vi "ThreadCfg - Read TxPkt Config.vi"(8 "error in (no error)":errorcluster, 11 "Node Ptr In":T4 format="%.0x") -> (0 "error out":errorcluster, 2 "threadOptions":T1 {"pclDecimation" max=16 step=1; "loopPeriod" max=16 step=1; "targetPriority" min=-2 max=16 step=1; "targetProcessor" min=-2 max=16 step=1}, 3 "Node Ptr Out":T4 format="%.0x")   [LabVIEW 2019, in "UDP-Custom-Device System Explorer.lvlib"]
uses:
  UDP-Custom-Device System Explorer.lvlib
  <vilib>/NI VeriStand/Custom Device API/Custom Device Item Ref.ctl
  Types/Threading/Thread Configuration.ctl
  Types/Threading/Thread Sync Reference.ctl
  Shared/Types/Shared - Thread Management.ctl
  Property Accessors/Tx Packet Accessors.lvlib
  Property Accessors/Shared Packet Accessors.lvlib
  Shared/UDP-Custom-Device Shared.lvlib
  <vilib>/NI VeriStand/Custom Device API/Custom Device API.lvlib
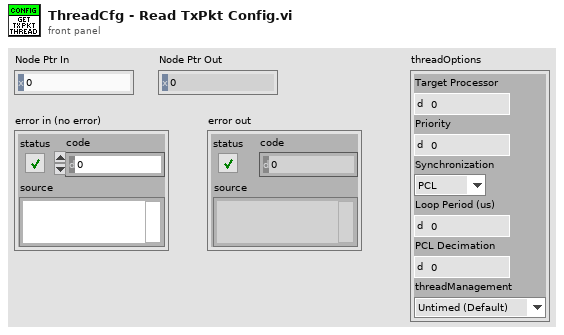
[diagram p1: front panel]
types:
  T1 = typedef "UDP-Custom-Device System Explorer.lvlib/Thread Configuration.ctl" = cluster{"targetProcessor":i8, "targetPriority":i16, "Synchronization":T2, "loopPeriod":u32, "pclDecimation":u16, "threadManagement":T3}
  T2 = typedef "UDP-Custom-Device System Explorer.lvlib/Thread Sync Reference.ctl" = enum16{"PCL", "Async"}
  T3 = typedef "UDP-Custom-Device Shared.lvlib/Shared - Thread Management.ctl" = enum16{"Untimed (Default)", "Timed (High Priority)"}
  T4 = typedef "Custom Device API.lvlib/Custom Device Item Ref.ctl" = u64
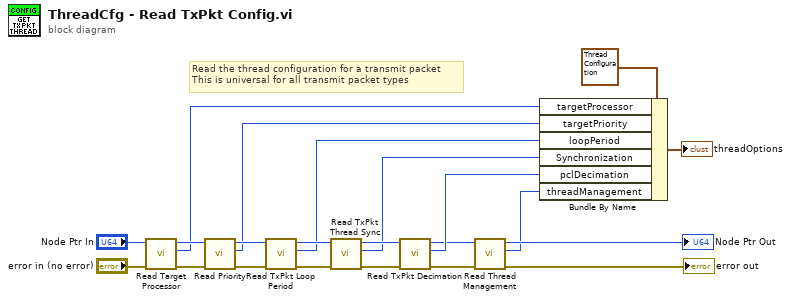
[diagram p0: block diagram]
diagram:
  # "Read the thread configuration for a transmit packet\nThis is universal for all transmit packet types"
  n1 = call "Read Target Processor.vi"("error in (no error)"="error in (no error)", "Node Ptr"="Node Ptr In") -> ("error out"=w19:errorcluster, "targetProcessor"=w6:i8, "Node Ptr out"=w20:T4)  [unwired: 7 in]
  n2 = call "Read Priority.vi"("error in (no error)"=w19, "Node Ptr"=w20) -> ("error out"=w17:errorcluster, "targetPriority"=w7:i16, "Node Ptr out"=w18:T4)  [unwired: 7 in]
  n3 = call "Read TxPkt Loop Period.vi"("error in (no error)"=w17, "Node Ptr"=w18) -> ("error out"=w16:errorcluster, "loopPeriod"=w8:u32, "Node Ptr out"=w15:T4)  [unwired: 7 in]
  n4 = call "Read TxPkt Thread Sync.vi"("error in (no error)"=w16, "Node Ptr"=w15) -> ("error out"=w13:errorcluster, "threadSync"=w9:T2, "Node Ptr out"=w14:T4)  [unwired: 7 in]
  n5 = call "Read TxPkt Decimation.vi"("error in (no error)"=w13, "Node Ptr"=w14) -> ("error out"=w3:errorcluster, "Decimation"=w10:u16, "Node Ptr out"=w5:T4)  [unwired: 7 in]
  n6 = call "Read Thread Management.vi"("error in (no error)"=w3, "Node Ptr"=w5) -> ("error out"=→"error out":errorcluster, "Thread Management"=w1:T3, "Node Ptr out"=→"Node Ptr Out":T4)  [unwired: 7 in]
  n7 = Bundle By Name(cluster=T1 {"targetProcessor"=0, "targetPriority"=0, "Synchronization"=enum."PCL", "loopPeriod"=0, "pclDecimation"=0, "threadManagement"=enum."Untimed (Default)"} ("threadOptions"), "targetProcessor"=w6, "targetPriority"=w7, "loopPeriod"=w8, "Synchronization"=w9, "pclDecimation"=w10, "threadManagement"=w1) -> (→"threadOptions":T1)
